vi "SVL AC & DC Level (Frequency) (1 Ch).vi"(0 "complex spectrum":T7 {"spectrum info"."x-axis units" items=["Time (s)"=0, "Frequency-CB (Hz)"=1, "Frequency-CPB (Hz)"=1248, "Frequency-Arbitrary (Hz)"=2357, "Quefrency (s)"=2, "Revolutions (rev)"=3, "Order"=4, "Speed (RPM)"=11, "Speed (rad/s)"=21, "Index"=65535]; "spectrum info"."weighting filter" items=["Linear", "A-weighting", "B-weighting", "C-weighting", "ITU-R 468-4", "Dolby", "CCITT", "C-message", "Wb", "Wc", "Wd", "We", "Wf", "Wh", "Wj", "Wk", "Wm", "AES17 20 kHz lowpass", "AES17 40 kHz lowpass", "AES17 20 kHz highpass", "AES17 40 kHz highpass"]; "spectrum info"."dB reference [EU]" format="%.2f"; "spectrum info"."engineering units" items=["custom..."=0, "V"=1, "A"=21, "C"=30, "pC"=31, "s"=32, "-"=29, "Pa"=2, "N"=20, "g"=3, "m/s^2"=4, "m/s"=5, "m"=6, "mm/s"=12, "mm"=13, "micron/s"=14, "micron"=15, "in/s^2"=7, "in/s"=8, "in"=9, "mil/s"=10, "mil"=11, "rad/s^2"=16, "rad/s"=17, "rad"=18, "deg/s^2"=26, "deg/s"=27, "deg"=28, "RPM"=22, "cycle/s^2"=23, "Hz"=24, "cycle"=25, "strain"=19]; "spectrum info"."spectral info"."window" items=["None "=0, "Hanning"=1, "Hamming"=2, "Blackman-Harris"=3, "Exact Blackman"=4, "Blackman"=5, "Flat Top"=6, "4 Term B-Harris "=7, "7 Term B-Harris"=8, "Low Sidelobe"=9, "Force - Exponential"=10, "Gaussian"=62]}, 5 "error in (no error)":errorcluster) -> (12 "unit label":string, 14 "AC complex spectrum":T7 {"spectrum info"."x-axis units" items=["Time (s)"=0, "Frequency-CB (Hz)"=1, "Frequency-CPB (Hz)"=1248, "Frequency-Arbitrary (Hz)"=2357, "Quefrency (s)"=2, "Revolutions (rev)"=3, "Order"=4, "Speed (RPM)"=11, "Speed (rad/s)"=21, "Index"=65535]; "spectrum info"."weighting filter" items=["Linear", "A-weighting", "B-weighting", "C-weighting", "ITU-R 468-4", "Dolby", "CCITT", "C-message", "Wb", "Wc", "Wd", "We", "Wf", "Wh", "Wj", "Wk", "Wm", "AES17 20 kHz lowpass", "AES17 40 kHz lowpass", "AES17 20 kHz highpass", "AES17 40 kHz highpass"]; "spectrum info"."dB reference [EU]" format="%.2f"; "spectrum info"."engineering units" items=["custom..."=0, "V"=1, "A"=21, "C"=30, "pC"=31, "s"=32, "-"=29, "Pa"=2, "N"=20, "g"=3, "m/s^2"=4, "m/s"=5, "m"=6, "mm/s"=12, "mm"=13, "micron/s"=14, "micron"=15, "in/s^2"=7, "in/s"=8, "in"=9, "mil/s"=10, "mil"=11, "rad/s^2"=16, "rad/s"=17, "rad"=18, "deg/s^2"=26, "deg/s"=27, "deg"=28, "RPM"=22, "cycle/s^2"=23, "Hz"=24, "cycle"=25, "strain"=19]; "spectrum info"."spectral info"."window" items=["None "=0, "Hanning"=1, "Hamming"=2, "Blackman-Harris"=3, "Exact Blackman"=4, "Blackman"=5, "Flat Top"=6, "4 Term B-Harris "=7, "7 Term B-Harris"=8, "Low Sidelobe"=9, "Force - Exponential"=10, "Gaussian"=62]}, 15 "AC level [EU rms]":dbl, 16 "DC complex spectrum":T7 {"spectrum info"."x-axis units" items=["Time (s)"=0, "Frequency-CB (Hz)"=1, "Frequency-CPB (Hz)"=1248, "Frequency-Arbitrary (Hz)"=2357, "Quefrency (s)"=2, "Revolutions (rev)"=3, "Order"=4, "Speed (RPM)"=11, "Speed (rad/s)"=21, "Index"=65535]; "spectrum info"."weighting filter" items=["Linear", "A-weighting", "B-weighting", "C-weighting", "ITU-R 468-4", "Dolby", "CCITT", "C-message", "Wb", "Wc", "Wd", "We", "Wf", "Wh", "Wj", "Wk", "Wm", "AES17 20 kHz lowpass", "AES17 40 kHz lowpass", "AES17 20 kHz highpass", "AES17 40 kHz highpass"]; "spectrum info"."dB reference [EU]" format="%.2f"; "spectrum info"."engineering units" items=["custom..."=0, "V"=1, "A"=21, "C"=30, "pC"=31, "s"=32, "-"=29, "Pa"=2, "N"=20, "g"=3, "m/s^2"=4, "m/s"=5, "m"=6, "mm/s"=12, "mm"=13, "micron/s"=14, "micron"=15, "in/s^2"=7, "in/s"=8, "in"=9, "mil/s"=10, "mil"=11, "rad/s^2"=16, "rad/s"=17, "rad"=18, "deg/s^2"=26, "deg/s"=27, "deg"=28, "RPM"=22, "cycle/s^2"=23, "Hz"=24, "cycle"=25, "strain"=19]; "spectrum info"."spectral info"."window" items=["None "=0, "Hanning"=1, "Hamming"=2, "Blackman-Harris"=3, "Exact Blackman"=4, "Blackman"=5, "Flat Top"=6, "4 Term B-Harris "=7, "7 Term B-Harris"=8, "Low Sidelobe"=9, "Force - Exponential"=10, "Gaussian"=62]}, 17 "DC level [EU]":dbl, 19 "error out":errorcluster)   [LabVIEW 2017]
doc: "Computes the AC level and DC level of a signal. Wire data to the <B>scaled signal [EU]</B> input to determine the polymorphic instance to use or manually select the instance."
uses:
  <vilib>/addons/_NISVFA/_Shared subVIs/Controls/svc_Spectrum Info.ctl
  <vilib>/addons/_NISVFA/_Shared subVIs/Controls/svc_X-Axis Units.ctl
  <vilib>/addons/_NISVFA/_Shared subVIs/Controls/svc_Spectrum Type.ctl
  <vilib>/addons/_NISVFA/_Shared subVIs/Controls/svc_Engineering Units Text Ring.ctl
  <vilib>/addons/_NISVFA/_Shared subVIs/Controls/svc_Weighting Filter Text Ring.ctl
  <vilib>/addons/_NISVFA/_Shared subVIs/Controls/svc_Complimentary Spectrum Units.ctl
  <vilib>/Analysis/2dsp.llb/Real FFT.vi
  <vilib>/Analysis/baseanly.llb/Mean (DBL).vi
  <vilib>/Analysis/4window.llb/Force Window.vi
  <vilib>/Analysis/4window.llb/Force Window (DBL).vi
  <vilib>/Analysis/4window.llb/Exponential Window.vi
  <vilib>/Analysis/4window.llb/Exponential Window (DBL).vi
  <vilib>/Analysis/BLAS.llb/dznrm2 - Vector 2-Norm (CDB).vi
  <vilib>/Utility/error.llb/Error Cluster From Error Code.vi
  <vilib>/Analysis/0measdsp.llb/Scaled Time Domain Window.vi
  <vilib>/Analysis/0measdsp.llb/Scaled Time Domain Window (DBL).vi
  <vilib>/addons/_NISVFA/_Spectrum Processing/subVIs/svfa_Spectrum Info Window to windowTd Type Def.vi
  <vilib>/addons/_NISVFA/_Shared subVIs/Common/svc_Get Weighting Enum and Labels.vi
  <vilib>/addons/_NISVFA/_Shared subVIs/Common/svc_Unit Label Lexical Class.vi
  <vilib>/addons/_NISVFA/_Shared subVIs/Common/svc_Engineering Units to Unit Label.vi
  <vilib>/addons/_NISVFA/_Shared subVIs/Common/svc_Format Value (DBL).vi
  <vilib>/Analysis/NI_AALPro.lvlib
  <vilib>/Analysis/NI_AALBLAS.lvlib
  <vilib>/Analysis/NI_AALBase.lvlib
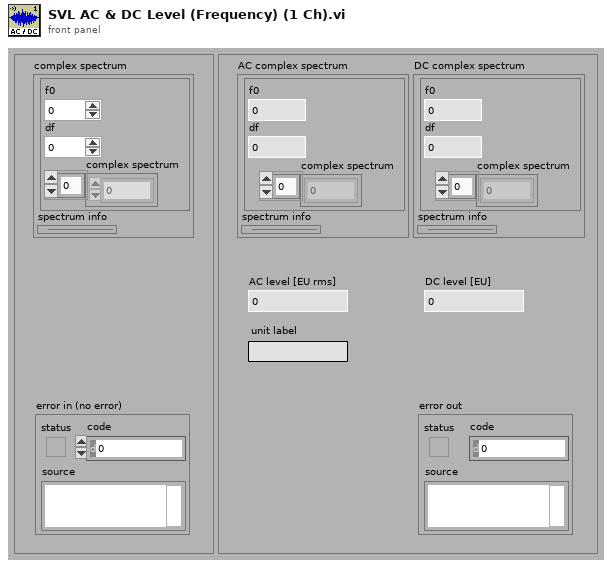
[diagram p1: front panel]
types:
  T1 = typedef "svc_Spectrum Info.ctl" = cluster{"channel name":string, "description":string, "x-axis units":T2, "spectral info":cluster{"spectrum type":T3, "linear/dB":enum16{"linear", "dB"}, "window":u16, "window size":i32, "FFT size":i32}, "engineering units":T4, "custom label":string, "dB reference [EU]":dbl, "peak units":enum16{"rms", "peak", "peak-peak"}, "weighting filter":T5, "spectral density?":bool, "unit label":string, "spectrum skewed?":bool, "complimentary spectrum units":T6}
  T2 = typedef "svc_X-Axis Units.ctl" = u16
  T3 = typedef "svc_Spectrum Type.ctl" = enum16{"FFT Spectrum [complex]", "Amplitude [Magnitude]", "Power [Magnitude^2]", "Cross Spectrum [complex]", "Frequency Response [Complex]"}
  T4 = typedef "svc_Engineering Units Text Ring.ctl" = u16
  T5 = typedef "svc_Weighting Filter Text Ring.ctl" = u16
  T6 = typedef "svc_Complimentary Spectrum Units.ctl" = enum16{"none", "radians", "degrees", "cycles", "imaginary"}
  T7 = cluster{"complex spectrum response":cluster{"f0":dbl, "df":dbl, "complex spectrum":cdb[]}, "spectrum info":T1}
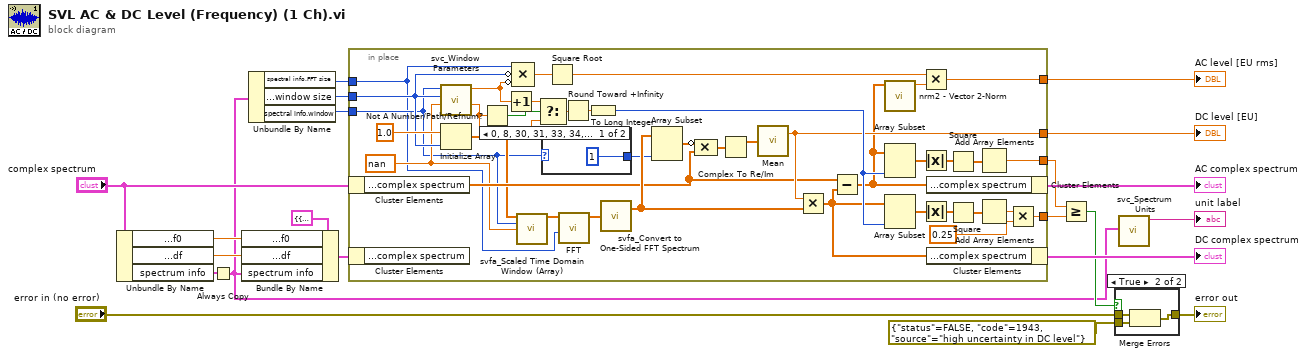
[diagram p0: block diagram]
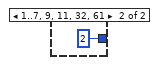
[diagram p2: hidden frame]
diagram:
  n1 = Unbundle By Name("complex spectrum") -> ("complex spectrum response.f0"=w11:dbl, "complex spectrum response.df"=w10:dbl, "spectrum info"=w5:T1)
  n2 = Always Copy(1:w5) -> (0:w1:T1)
  n3 = Bundle By Name(cluster=T7 {"complex spectrum response"={"f0"=0.0, "df"=1.0, "complex spectrum"=[]}, "spectrum info"={"channel name"="Channel0", "description"="", "x-axis units"=1, "spectral info"={"spectrum type"=enum."FFT Spectrum [complex]", "linear/dB"=enum."linear", "window"=1, "window size"=1000, "FFT size"=1000}, "engineering units"=0, "custom label"="EU", "dB reference [EU]"=1.0, "peak units"=enum."rms", "weighting filter"=0, "spectral density?"=FALSE, "unit label"="EU rms|SV Units|dB rms ref 1.0E+0 EU", "spectrum skewed?"=FALSE, "complimentary spectrum units"=enum."none"}} ("complex spectrum"), "complex spectrum response.f0"=w11, "complex spectrum response.df"=w10, "spectrum info"=w1) -> (w9:T7)
  n4 = Unbundle By Name(w1) -> ("spectral info.FFT size"=w14:i32, "spectral info.window size"=w3:i32, "spectral info.window"=w13:u16)
  n5 = in-place {
    in-place-border: [w23] -> w19
    in-place-border: [w46] -> w18
    in-place-border: w3 -> [w31]
    in-place-border: w14 -> [w22]
    in-place-border: w13 -> [w29]
    in-place-border: [w36] -> w8
    in-place-border: [w35] -> w7
    w30 = nan ("window parameter")
    n6 = in-place-cluster #1("complex spectrum") -> ("complex spectrum response.complex spectrum"=w38:cdb[])
    n7 = in-place-cluster #2(w9) -> ()  [unwired: 1 out]
    n8 = call <vilib>:"svc_Window Parameters.vi"("standard deviation"=w30, "window size"=w31, "window"=w29) -> ("6dB BW"=w57:dbl, "ENBW"=w39:dbl)  [unwired: 5 in, 2 out]
    n9 = Initialize Array(1.0 ("element"), w31) -> (w34:dbl[])
    n10 = Not A Number/Path/Refnum?(number/path/refnum=w57) -> (NaN/Path/Refnum?=w56:bool)
    n11 = Increment(x=w39) -> (x+1=w58:dbl)
    n12 = Compound Arithmetic op=MULTIPLY(w22, invert w31, invert w39) -> (w25:dbl)
    n13 = call <vilib>:"svfa_Scaled Time Domain Window (Array).vi"("input signal"=w34, "window"=w29, "window parameter"=w30) -> ("windowed signal"=w33:dbl[])  [unwired: 7 in, 5 out]
    n14 = Select(t=w58, s=w56, f=w57) -> (s? t:f=w59:dbl)
    n15 = case shown="0, 8, 30, 31, 33, 34, 60, 62, Default" w29 {
      tunnel: [1 ("length") 2 ("length")] -> w45
      frame 0, 8, 30, 31, 33, 34, 60, 62, Default {
      }
      frame 1..7, 9, 11, 32, 61 {
      }
    }
    n16 = Square Root(x=w25) -> (sqrt(x)=w24:dbl)
    n17 = call-poly <vilib>:"FFT.vi"("FFT size"=w22, "X"=w33) -> ("FFT {X}"=w41:cdb[])  [unwired: 8 in, 1 out]
    n18 = Round Toward +Infinity(x=w59) -> (ceil(x): smallest int >= x=w49:dbl)
    n19 = To Long Integer(number=w49) -> (32bit integer=w53:i32)
    n20 = call <vilib>:"svfa_Convert to One-Sided FFT Spectrum.vi"("two-sided FFT spectrum"=w41) -> ("one-sided FFT spectrum"=w47:cdb[])  [unwired: 1 out]
    n21 = Array Subset(array=w47, length=w45) -> (w42:cdb[])  [unwired: 1 in]
    n22 = Compound Arithmetic op=MULTIPLY(invert w42, w38) -> (w43:cdb[])
    n23 = Complex To Re/Im(x + iy=w43) -> (x=w44:dbl[])  [unwired: 1 out]
    n24 = call-poly <vilib>:"Mean.vi"("X"=w44) -> ("mean"=w46:dbl)  [unwired: 1 out]
    n25 = Multiply(x=w46, y=w47) -> (x*y=w37:cdb[])
    n26 = Subtract(x=w38, y=w37) -> (x-y=w28:cdb[])
    n27 = call-poly <vilib>:"nrm2 - Vector 2-Norm.vi"("x"=w28) -> ("dznrm2"=w26:dbl)  [unwired: 9 in, 1 out]
    n28 = Array Subset(array=w28, length=w53) -> (w51:cdb[])  [unwired: 1 in]
    n29 = Array Subset(array=w37, length=w53) -> (w50:cdb[])  [unwired: 1 in]
    n30 = Multiply(x=w24, y=w26) -> (x*y=w23:dbl)
    n31 = Absolute Value(x=w51) -> (abs(x)=w32:dbl[])
    n32 = Absolute Value(x=w50) -> (abs(x)=w54:dbl[])
    n33 = in-place-cluster #1("complex spectrum response.complex spectrum"=w28) -> (→"AC complex spectrum":T7)
    n34 = in-place-cluster #2("complex spectrum response.complex spectrum"=w37) -> (→"DC complex spectrum":T7)
    n35 = Square(x=w32) -> (x^2=w27:dbl[])
    n36 = Square(x=w54) -> (x^2=w48:dbl[])
    n37 = Add Array Elements(numeric array=w27) -> (sum=w36:dbl)
    n38 = Add Array Elements(numeric array=w48) -> (sum=w52:dbl)
    n39 = Multiply(x=w52, y=0.25) -> (x*y=w35:dbl)
  }
  "AC level [EU rms]" <- w19
  "DC level [EU]" <- w18
  n40 = Greater Or Equal?(x=w8, y=w7) -> (x >= y?=w6:bool)
  n41 = case shown="True" w6 {
    tunnel: "error in (no error)" -> [w62 w65]
    tunnel: [w62 w64] -> w21
    tunnel: errorcluster {"status"=FALSE, "code"=1943, "source"="high uncertainty in DC level"} ("error in 2 (no error)") -> [_ w63]
    frame False {
    }
    frame True {
      n42 = Merge Errors(w65, w63) -> (w64:errorcluster)
    }
  }
  "error out" <- w21
  n43 = call <vilib>:"svc_Spectrum Units.vi"("spectrum info in"=w1) -> ("unit label"=→"unit label":string)  [unwired: 3 in, 3 out]
